vi "Merge Async VI Error.vi"(8 "error in (no error)":errorcluster) -> (0 "error out":errorcluster)   [LabVIEW 2025, in "I2C Bus Monitor UI.lvlib"]
uses:
  I2C Bus Monitor UI.lvlib
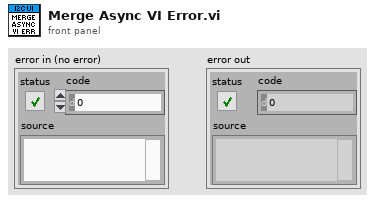
[diagram p1: front panel]
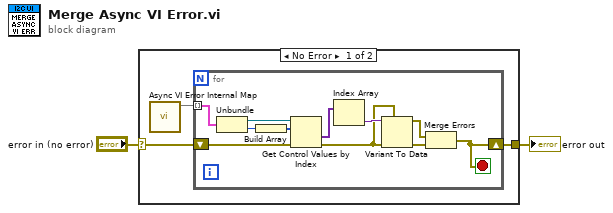
[diagram p0: block diagram]
diagram:
  n1 = case shown="No Error" "error in (no error)" {
    selector: "error in (no error)" -> [w4 w17]
    tunnel: [w3 w17] -> w1
    frame No Error {
      n2 = call "Async VI Error Internal Map.vi"() -> ("Error Out Indices Map out"=w5:map{refnum<vi>, i32})  [unwired: 11 in]
      n3 = for {
        tunnel: w5 -> [w15] mode=indexing
        shift-right: [w7] -> w3
        shift-left: w4 -> [w16]
        stop <- w7 stop-if-true
        n4 = Unbundle(w15) -> ("VI Ref"=w14:refnum<vi>, "ControlIndex"=w13:i32)
        n5 = Build Array(w13) -> (w12:i32[])
        n6 = Get Control Values by Index(0:w14, 1:w12, 3:w16) -> (10:w11:variant[], 11:w9:errorcluster)
        n7 = Index Array(array=w11) -> (element=w10:variant)  [unwired: 1 in]
        n8 = Variant To Data(error in=w9, type=w9, Variant=w10) -> (data=w6:errorcluster, error out=w8:errorcluster)
        n9 = Merge Errors(w6, w8) -> (w7:errorcluster)
      }
    }
    frame Error {
    }
  }
  "error out" <- w1
